vi "探头型号.vi"(11 "校准参数":u16(ring) caption="校准参数：" items=["pH", "DO", "浊度", "电导率", "叶绿素a", "藻密度", "ORP", "DO2"]) -> (3 "探头型号":u16(ring)=2 items=["禹山", "国弘", "纳清"], 5 "禁用项[]":i32[](array[numeric]), 7 "value":i32)   [LabVIEW 2016, in "斯坦道多参数.lvlib"]
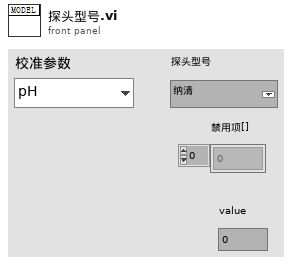
[diagram p1: front panel]
types:
  T1 = cluster{"pH探头选择":u16, "DO探头选择":u16, "电导率探头选择":u16, "浊度探头选择":u16, "叶绿素a探头选择":u16, "蓝绿藻探头选择":u16, "orp探头选择":u16, "COD探头选择":u16, "DO2探头选择":u16}
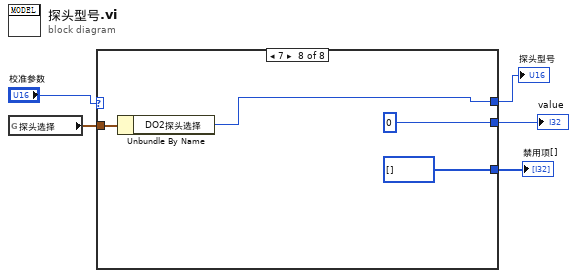
[diagram p0: block diagram]
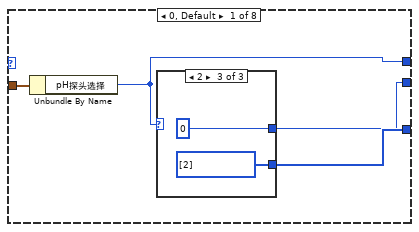
[diagram p2: hidden frame]
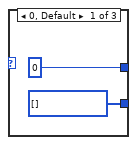
[diagram p3: hidden frame]
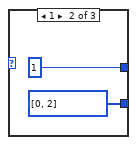
[diagram p4: hidden frame]
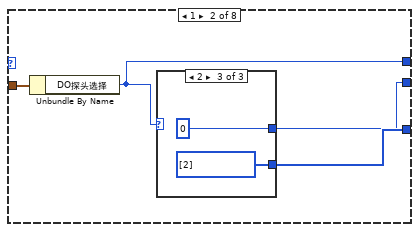
[diagram p5: hidden frame]
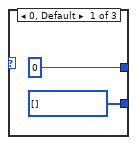
[diagram p6: hidden frame]
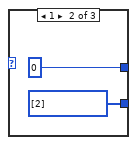
[diagram p7: hidden frame]
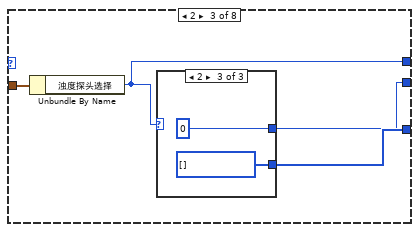
[diagram p8: hidden frame]
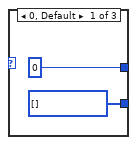
[diagram p9: hidden frame]
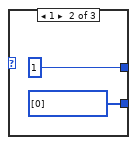
[diagram p10: hidden frame]
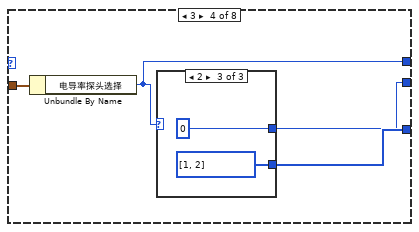
[diagram p11: hidden frame]
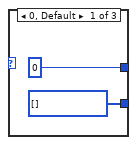
[diagram p12: hidden frame]
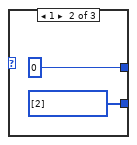
[diagram p13: hidden frame]
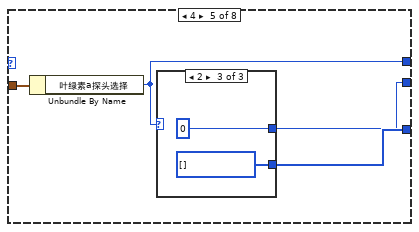
[diagram p14: hidden frame]
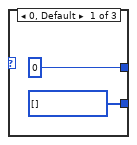
[diagram p15: hidden frame]
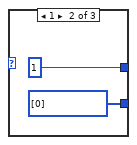
[diagram p16: hidden frame]
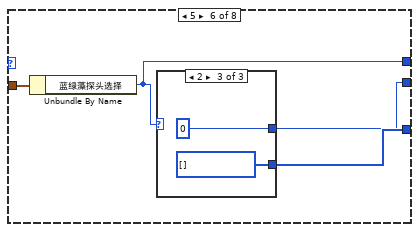
[diagram p17: hidden frame]
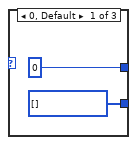
[diagram p18: hidden frame]
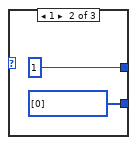
[diagram p19: hidden frame]
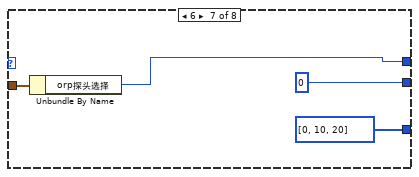
[diagram p20: hidden frame]
diagram:
  n1 = global read "断电保存变量.vi" "探头选择"() -> (w4:T1)
  n2 = case shown="7" "校准参数" {
    tunnel: w4 -> [w9 w19 w29 w39 w49 w59 w69 w73]
    tunnel: [w8 w18 w28 w38 w48 w58 w68 w72] -> w3
    tunnel: [w7 w17 w27 w37 w47 w57 i32[] [0, 10, 20] ("禁用项[]") i32[] [] ("禁用项[]")] -> w2
    tunnel: [w6 w16 w26 w36 w46 w56 0 0] -> w1
    frame 0, Default {
      n3 = Unbundle By Name(w9) -> ("pH探头选择"=w8:u16)
      n4 = case shown="2" w8 {
        tunnel: [i32[] [] ("禁用项[]") i32[] [0, 2] ("禁用项[]") i32[] [2] ("禁用项[]")] -> w7
        tunnel: [0 1 0] -> w6
        frame 0, Default {
        }
        frame 1 {
        }
        frame 2 {
        }
      }
    }
    frame 1 {
      n5 = Unbundle By Name(w19) -> ("DO探头选择"=w18:u16)
      n6 = case shown="2" w18 {
        tunnel: [i32[] [] ("禁用项[]") i32[] [2] ("禁用项[]") i32[] [2] ("禁用项[]")] -> w17
        tunnel: [0 0 0] -> w16
        frame 0, Default {
        }
        frame 1 {
        }
        frame 2 {
        }
      }
    }
    frame 2 {
      n7 = Unbundle By Name(w29) -> ("浊度探头选择"=w28:u16)
      n8 = case shown="2" w28 {
        tunnel: [i32[] [] ("禁用项[]") i32[] [0] ("禁用项[]") i32[] [] ("禁用项[]")] -> w27
        tunnel: [0 1 0] -> w26
        frame 0, Default {
        }
        frame 1 {
        }
        frame 2 {
        }
      }
    }
    frame 3 {
      n9 = Unbundle By Name(w39) -> ("电导率探头选择"=w38:u16)
      n10 = case shown="2" w38 {
        tunnel: [i32[] [] ("禁用项[]") i32[] [2] ("禁用项[]") i32[] [1, 2] ("禁用项[]")] -> w37
        tunnel: [0 0 0] -> w36
        frame 0, Default {
        }
        frame 1 {
        }
        frame 2 {
        }
      }
    }
    frame 4 {
      n11 = Unbundle By Name(w49) -> ("叶绿素a探头选择"=w48:u16)
      n12 = case shown="2" w48 {
        tunnel: [i32[] [] ("禁用项[]") i32[] [0] ("禁用项[]") i32[] [] ("禁用项[]")] -> w47
        tunnel: [0 1 0] -> w46
        frame 0, Default {
        }
        frame 1 {
        }
        frame 2 {
        }
      }
    }
    frame 5 {
      n13 = Unbundle By Name(w59) -> ("蓝绿藻探头选择"=w58:u16)
      n14 = case shown="2" w58 {
        tunnel: [i32[] [] ("禁用项[]") i32[] [0] ("禁用项[]") i32[] [] ("禁用项[]")] -> w57
        tunnel: [0 1 0] -> w56
        frame 0, Default {
        }
        frame 1 {
        }
        frame 2 {
        }
      }
    }
    frame 6 {
      n15 = Unbundle By Name(w69) -> ("orp探头选择"=w68:u16)
    }
    frame 7 {
      n16 = Unbundle By Name(w73) -> ("DO2探头选择"=w72:u16)
    }
  }
  "探头型号" <- w3
  "禁用项[]" <- w2
  "value" <- w1
